vi "Valid Answers--constant.vi"() -> (2 "Valid Answers Array":string[](array[string]), 3 "Valid Answers Set":set{string}(c389))   [LabVIEW 2020, in "Wordle Engine.lvlib"]
uses:
  Wordle Engine.lvlib
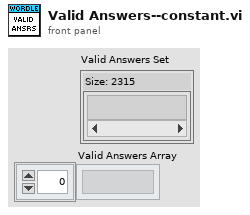
[diagram p1: front panel]
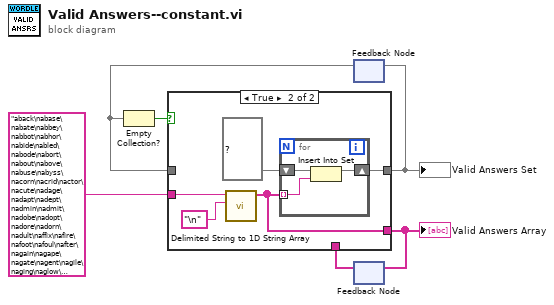
[diagram p0: block diagram]
diagram:
  n1 = feedback #1() -> (w4:set{string})  [unwired: 1 in]
  n2 = Empty Collection?(1:w4) -> (0:w6:bool)
  n3 = feedback #2() -> (w1:string[])  [unwired: 1 in]
  n4 = case shown="True" w6 {
    tunnel: "aback\nabase\nabate\nabbey\nabbot\nabhor\nabide\nabled\nabode\nabort\nabout\nabove\nabuse\nabyss\nacorn\nacrid\nactor\nacute\nadage\nadapt\nadept\nadmin\nadmit\nadobe\nadopt\nadore\nadorn\nadult\naffix\nafire\nafoot\nafoul\nafter\nagain\nagape\nagate\nagent\nagile\naging\naglow\nagony\nagora\nagree\nahead\naider\naisle\nalarm\nalbum\nalert\nalgae\nalibi\nalien\nalign\nalike\nalive\nallay\nalley\nallot\nallow\nalloy\naloft\nalone\nalong\naloof\naloud\nalpha\naltar\nalter\namass\namaze\namber\namble\namend\namiss\namity\namong\nample\namply\namuse\nangel\nanger\nangle\nangry\nangst\nanime\nankle\nannex\nannoy\nannul\nanode\nantic\nanvil\naorta\napart\naphid\naping\napnea\napple\napply\napron\n..." -> [_ w13]
    tunnel: [w8 w11] -> w3
    tunnel: w4 -> [w8 _]
    tunnel: [w7 w9] -> w2
    tunnel: w1 -> [w7 _]
    frame False {
    }
    frame True {
      n5 = call <vilib>:"Delimited String to 1D String Array.vi"("delimiter"="\n", "delimited string"=w13) -> ("string array"=w9:string[])  [unwired: 9 in]
      n6 = for {
        tunnel: w9 -> [w14] mode=indexing
        shift-right: [w16] -> w11
        shift-left: set{string} {} ("Valid Guesses") -> [w15]
        n7 = Insert Into Set(10:w14, 11:w15) -> (3:w16:set{string})  [unwired: 1 out]
      }
    }
  }
  "Valid Answers Set" <- w3
  "Valid Answers Array" <- w2
  n8 = feedback-in #1(w3) -> ()
  n9 = feedback-in #2(w2) -> ()
